vi "Timer.vi"(10 "Time Target":dbl, 11 "Last iteration Time":timestamp) -> (3 "Time Elapsed?":bool)   [LabVIEW 2024]
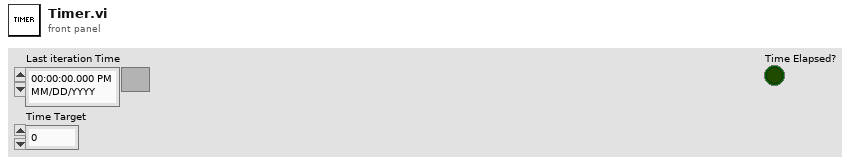
[diagram p1: front panel]
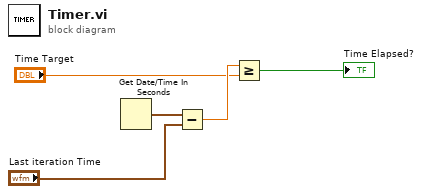
[diagram p0: block diagram]
diagram:
  n1 = Get Date/Time In Seconds() -> (seconds since 1Jan1904=w2:timestamp)
  n2 = Subtract(x=w2, y="Last iteration Time") -> (x-y=w5:dbl)
  n3 = Greater Or Equal?(x=w5, y="Time Target") -> (x >= y?=→"Time Elapsed?":bool)
